vi "Script Work CBR.vi"(4 "Special Terminals":T1={"Action"=-1, "Init"=-1, "Tag"=-1, "State in"=-1, "State out"=-1, "Error"=-1}, 6 "Terminal Configs":T2[](array[typedef]), 8 "error in (no error)":errorcluster, 11 "Refs in":T8) -> (0 "error out":errorcluster, 3 "Refs":T8)   [LabVIEW 2020, in "FlexBlocks.lvlib"]
uses:
  FlexBlocks.lvlib
  Scripting Refs.ctl
  Terminal Config.ctl
  Type Descriptor.ctl
  Terminal Direction.ctl
  Value Mode.ctl
  Special Terminal.ctl
  Terminal Mode.ctl
  Special Terminal Indices.ctl
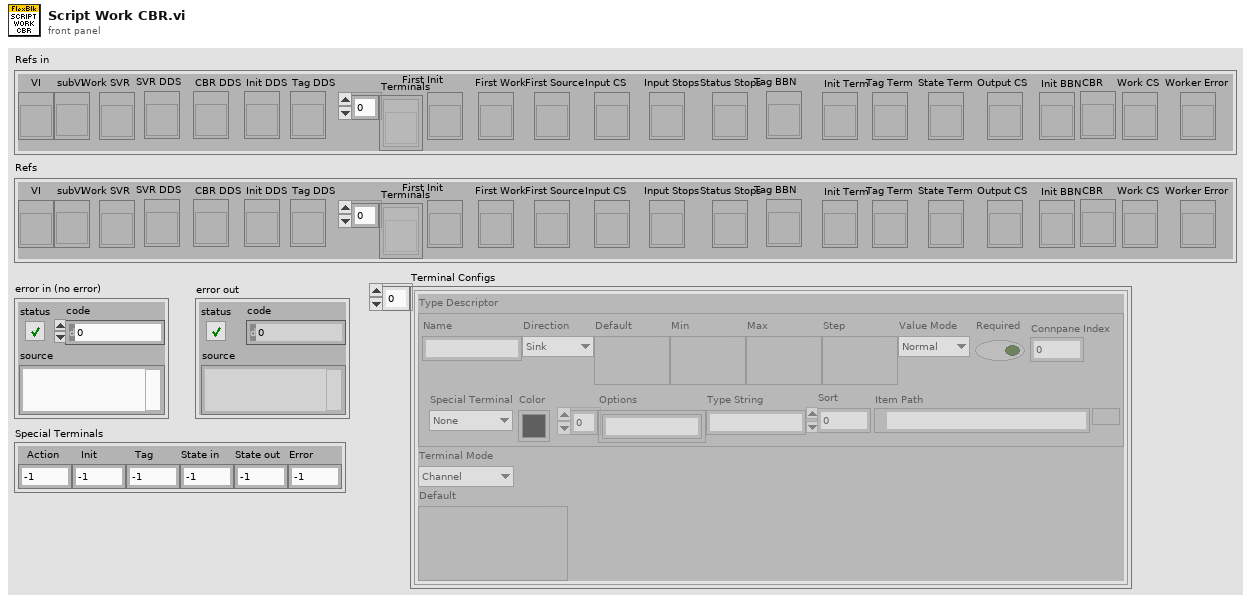
[diagram p1: front panel]
types:
  T1 = typedef "FlexBlocks.lvlib/Special Terminal Indices.ctl" = cluster{"Action":i32, "Init":i32, "Tag":i32, "State in":i32, "State out":i32, "Error":i32}
  T2 = typedef "FlexBlocks.lvlib/Terminal Config.ctl" = cluster{"Type Descriptor":T3, "Terminal Mode":T7, "Default":variant}
  T3 = typedef "FlexBlocks.lvlib/Type Descriptor.ctl" = cluster{"Name":string, "Direction":T4, "Default":variant, "Min":variant, "Max":variant, "Step":variant, "Value Mode":T5, "Required":bool, "Connpane Index":i32, "Special Terminal":T6, "Color":u32, "Options":string[], "Type String":string, "Sort":i32, "Item Path":path}
  T4 = typedef "FlexBlocks.lvlib/Terminal Direction.ctl" = enum16{"Sink", "Source"}
  T5 = typedef "FlexBlocks.lvlib/Value Mode.ctl" = enum16{"Normal", "Range", "Select"}
  T6 = typedef "FlexBlocks.lvlib/Special Terminal.ctl" = enum16{"None", "Action", "Init", "Tag", "State in", "State out", "Error"}
  T7 = typedef "FlexBlocks.lvlib/Terminal Mode.ctl" = enum16{"Channel", "Config", "Value", "Control Ref"}
  T8 = typedef "FlexBlocks.lvlib/Scripting Refs.ctl" = cluster{"VI":refnum<vi>, "subVI":refnum<vi>, "Work SVR":refnum<vi>, "SVR DDS":refnum<vi>, "CBR DDS":refnum<vi>, "Init DDS":refnum<vi>, "Tag DDS":refnum<vi>, "Terminals":refnum<vi>[], "First Init":refnum<vi>, "First Work":refnum<vi>, "First Source":refnum<vi>, "Input CS":refnum<vi>, "Input Stops":refnum<vi>, "Status Stops":refnum<vi>, "Tag BBN":refnum<vi>, "Init Term":refnum<vi>, "Tag Term":refnum<vi>, "State Term":refnum<vi>, "Output CS":refnum<vi>, "Init BBN":refnum<vi>, "CBR":refnum<vi>, "Work CS":refnum<vi>, "Worker Error":refnum<vi>}
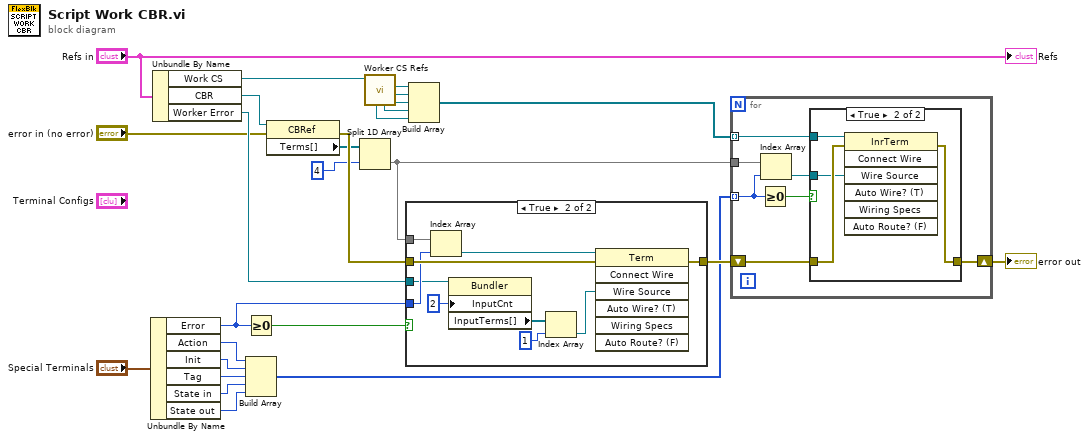
[diagram p0: block diagram]
diagram:
  n1 = Unbundle By Name("Special Terminals") -> ("Error"=w1:i32, "Action"=w15:i32, "Init"=w16:i32, "Tag"=w17:i32, "State in"=w14:i32, "State out"=w13:i32)
  n2 = Unbundle By Name("Refs in") -> ("Work CS"=w24:refnum<vi>, "CBR"=w22:refnum<vi>, "Worker Error"=w19:refnum<vi>)
  n3 = Greater Or Equal To 0?(x=w1) -> (x >= 0?=w23:bool)
  n4 = Build Array(w15, w16, w17, w14, w13) -> (w6:i32[])
  n5 = property class="CBRef"(reference=w22, error in="error in (no error)") -> (error out=w26:errorcluster, "Terms[]"=w21:refnum<vi>[])  [unwired: 1 out]
  n6 = Split 1D Array(array=w21, index=4) -> (second subarray=w4:refnum<vi>[])  [unwired: 1 out]
  n7 = call "Worker CS Refs.vi"("Work CS in"=w24) -> ("Tag In"=w10:refnum<vi>, "Init In"=w11:refnum<vi>, "Action In"=w12:refnum<vi>, "State In"=w9:refnum<vi>, "State Out"=w8:refnum<vi>)  [unwired: 5 in, 1 out]
  n8 = case shown="True" w23 {
    tunnel: w1 -> [_ w35]
    tunnel: w4 -> [_ w36]
    tunnel: w19 -> [_ w34]
    tunnel: [w27 w28] -> w7
    tunnel: w26 -> [w27 w37]
    frame False {
    }
    frame True {
      n9 = Index Array(array=w36, index=w35) -> (element=w30:refnum<vi>)
      n10 = property class="Bundler"(reference=w34, "InputCnt"=2 ("Input Count")) -> ("InputTerms[]"=w32:refnum<vi>[])  [unwired: 1 in, 2 out]
      n11 = Index Array(array=w32, index=1) -> (element=w29:refnum<vi>)
      n12 = invoke class="Term" method="Connect Wire"(reference=w30, error in=w37, "Wire Source"=w29) -> (error out=w28:errorcluster)  [unwired: 4 in, 6 out]
    }
  }
  n13 = Build Array(w12, w11, w10, w9, w8) -> (w5:refnum<vi>[])
  n14 = for {
    shift-right: [w40] -> w2
    shift-left: w7 -> [w41]
    tunnel: w6 -> [w43] mode=indexing
    tunnel: w5 -> [w38] mode=indexing
    tunnel: w4 -> [w44]
    n15 = Greater Or Equal To 0?(x=w43) -> (x >= 0?=w42:bool)
    n16 = Index Array(array=w44, index=w43) -> (element=w39:refnum<vi>)
    n17 = case shown="True" w42 {
      tunnel: w41 -> [w45 w48]
      tunnel: [w45 w46] -> w40
      tunnel: w39 -> [_ w47]
      tunnel: w38 -> [_ w49]
      frame False {
      }
      frame True {
        n18 = invoke class="InrTerm" method="Connect Wire"(reference=w49, error in=w48, "Wire Source"=w47) -> (error out=w46:errorcluster)  [unwired: 4 in, 6 out]
      }
    }
  }
  "error out" <- w2
  "Refs" <- "Refs in"
